vi "cBRS Readout Transfer Function.vi"() -> ()   [LabVIEW 2018]
uses:
  <vilib>/Utility/error.llb/DialogType.ctl
  <vilib>/DAQmx/read.llb/DAQmx Read (Analog 1D Wfm NChan NSamp).vi
  <vilib>/DAQmx/write.llb/DAQmx Write (Analog DBL 1Chan 1Samp).vi
  <vilib>/DAQmx/create/channels.llb/DAQmx Create Channel (AI-Voltage-Basic).vi
  <vilib>/DAQmx/configure/timing.llb/DAQmx Timing (Sample Clock).vi
  <vilib>/DAQmx/create/channels.llb/DAQmx Create Channel (AO-Voltage-Basic).vi
  <vilib>/DAQmx/miscellaneous.llb/DAQmx Fill In Error Info.vi
panel:
  in  "Amplitude":dbl=7.0
  in  "Frequency":dbl
  in  "Capacitor Feedback":bool
  in  "Piezo Feedback":bool
  in  "Gain 1":dbl
  in  "Physical Channel 5":tag="Dev1/ao3" caption="Physical Channel"
  in  "Physical Channel 4":tag="Dev1/ao2" caption="Physical Channel"
  in  "I Reset 2":bool
  in  "I Reset 1":bool
  in  "To Disk Freq":dbl=500.0 caption="dt"
  in  "DC Offset 2":dbl
  in  "I term 2":dbl=5000.0
  in  "Gain 2":dbl=0.005
  in  "Setpoint 2":dbl=5.0
  in  "Physical Channel 3":tag="Dev1/ao1" caption="Physical Channel"
  in  "I term":dbl=5000.0
  in  "Output terminal configuration":i32(ring)=10083 items=["Default"=-1, "RSE"=10083, "Differential"=10106, "Pseudodifferential"=12529]
  in  "DC Offset":dbl
  in  "Gain":dbl=0.005
  in  "Setpoint":dbl=5.0
  in  "Physical Channel 2":tag="Dev1/ao0" caption="Physical Channel"
  in  "Input terminal configuration":i32(ring)=10106 items=["default"=-1, "RSE"=10083, "NRSE"=10078, "Differential"=10106, "Pseudodifferential"=12529]
  in  "Down Sample Freq":dbl=1000.0 caption="dt"
  out "Waveform Chart":dynamicdata(graph)=[{"t0"=timestamp(3662756182.4372287 s since 1904-01-01), "dt"=1.9999999999999998e-05, "Y"=array[500 elements], "attributes"=variant("NI_ChannelName"=variant(string "Dev1/ai0"), "NI_UnitDescription"=variant(string "Volts"))}, {"t0"=timestamp(3662756182.4372387 s since 1904-01-01), "dt"=1.9999999999999998e-05, "Y"=array[500 elements], "attributes"=variant("NI_ChannelName"=variant(string "Dev1/ai2"), "NI_UnitDescription"=variant(string "Volts"))}, {"t0"=timestamp(3662756182.4372287 s since 1904-01-01), "dt"=0.001, "Y"=[0.0, 0.0, 0.0, 0.0, 0.0, 0.0, 0.0, 0.0, 0.0, 0.0], "attributes"=variant("NI_ChannelName"=variant(string "Dev1/ai0 (Filtered)"), "NI_OriginalChannelName"=variant(string "Dev1/ai0"), "NI_UnitDescription"=variant(string "Volts"))}, {"t0"=timestamp(3662756182.4372287 s since 1904-01-01), "dt"=0.001, "Y"=[0.0, 0.0, 0.0, 0.0, 0.0, 0.0, 0.0, 0.0, 0.0, 0.0], "attributes"=variant("NI_ChannelName"=variant(string "Dev1/ai2 (Filtered)"), "NI_OriginalChannelName"=variant(string "Dev1/ai2"), "NI_UnitDescription"=variant(string "Volts"))}, {"t0"=timestamp(3662756182.4372287 s since 1904-01-01), "dt"=0.001, "Y"=[3.746254926547408, 3.7462550457566977, 3.7462551556527615, 3.746255255304277, 3.7462553502991796, 3.746255445294082, 3.7462555365636945, 3.7462556241080165, 3.7462557135149837, 3.7462558085098863], "attributes"=variant("NI_ChannelName"=variant(string "Dev1/ai0 (Filtered)"), "NI_OriginalChannelName"=variant(string "Dev1/ai0"), "NI_UnitDescription"=variant(string "Volts"))}]
  in  "Write":bool caption="Enable"
  in  "stop":bool
  in  "Samples to Read":i32=500
  in  "Sample Rate":dbl=50000.0 caption="Read Rate (Hz)" format="%0.2f"
  in  "Physical Channel":tag="Dev1/ai0, Dev1/ai2" caption="Input Physical Channel"
  # "Piezo Feedback 1"
  # "Piezo Feedback 2"
  # "Capacitor Feedback"
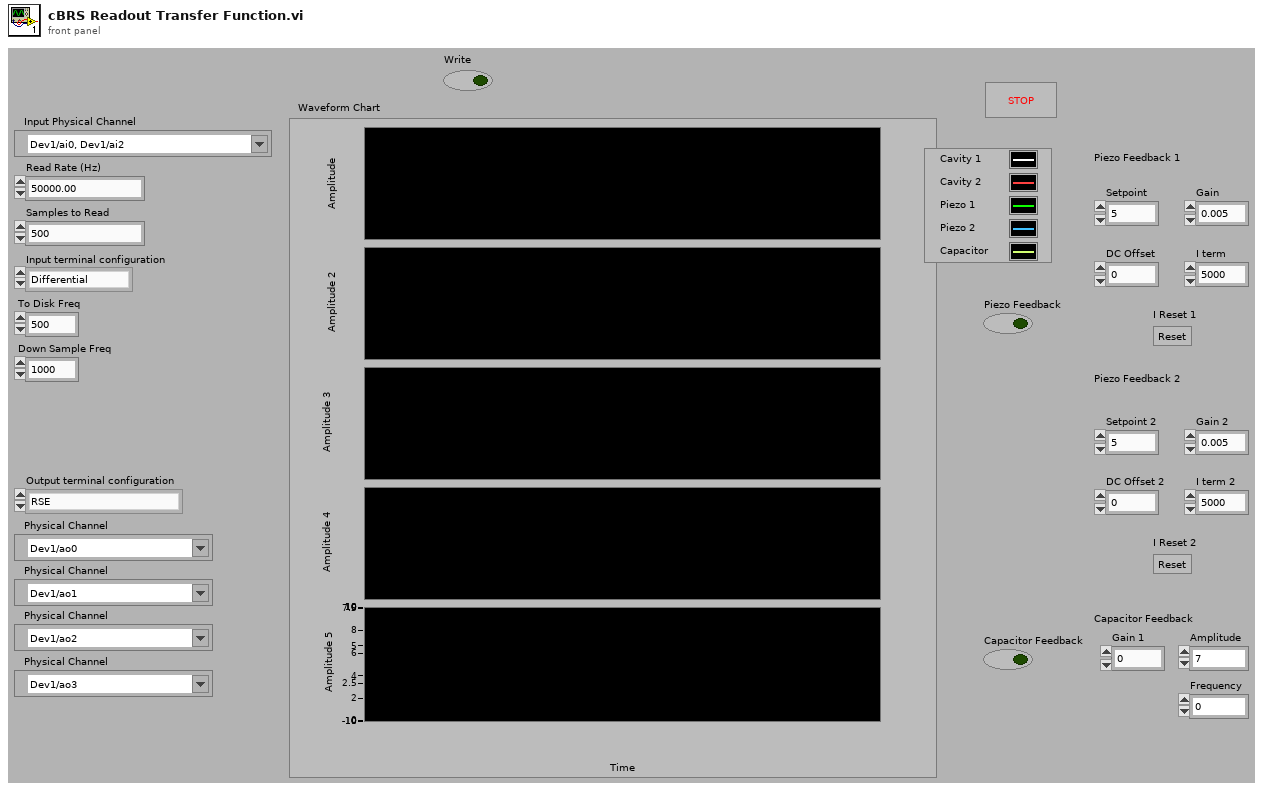
[diagram p1: front panel]
types:
  T1 = typedef "DialogType.ctl" = u16
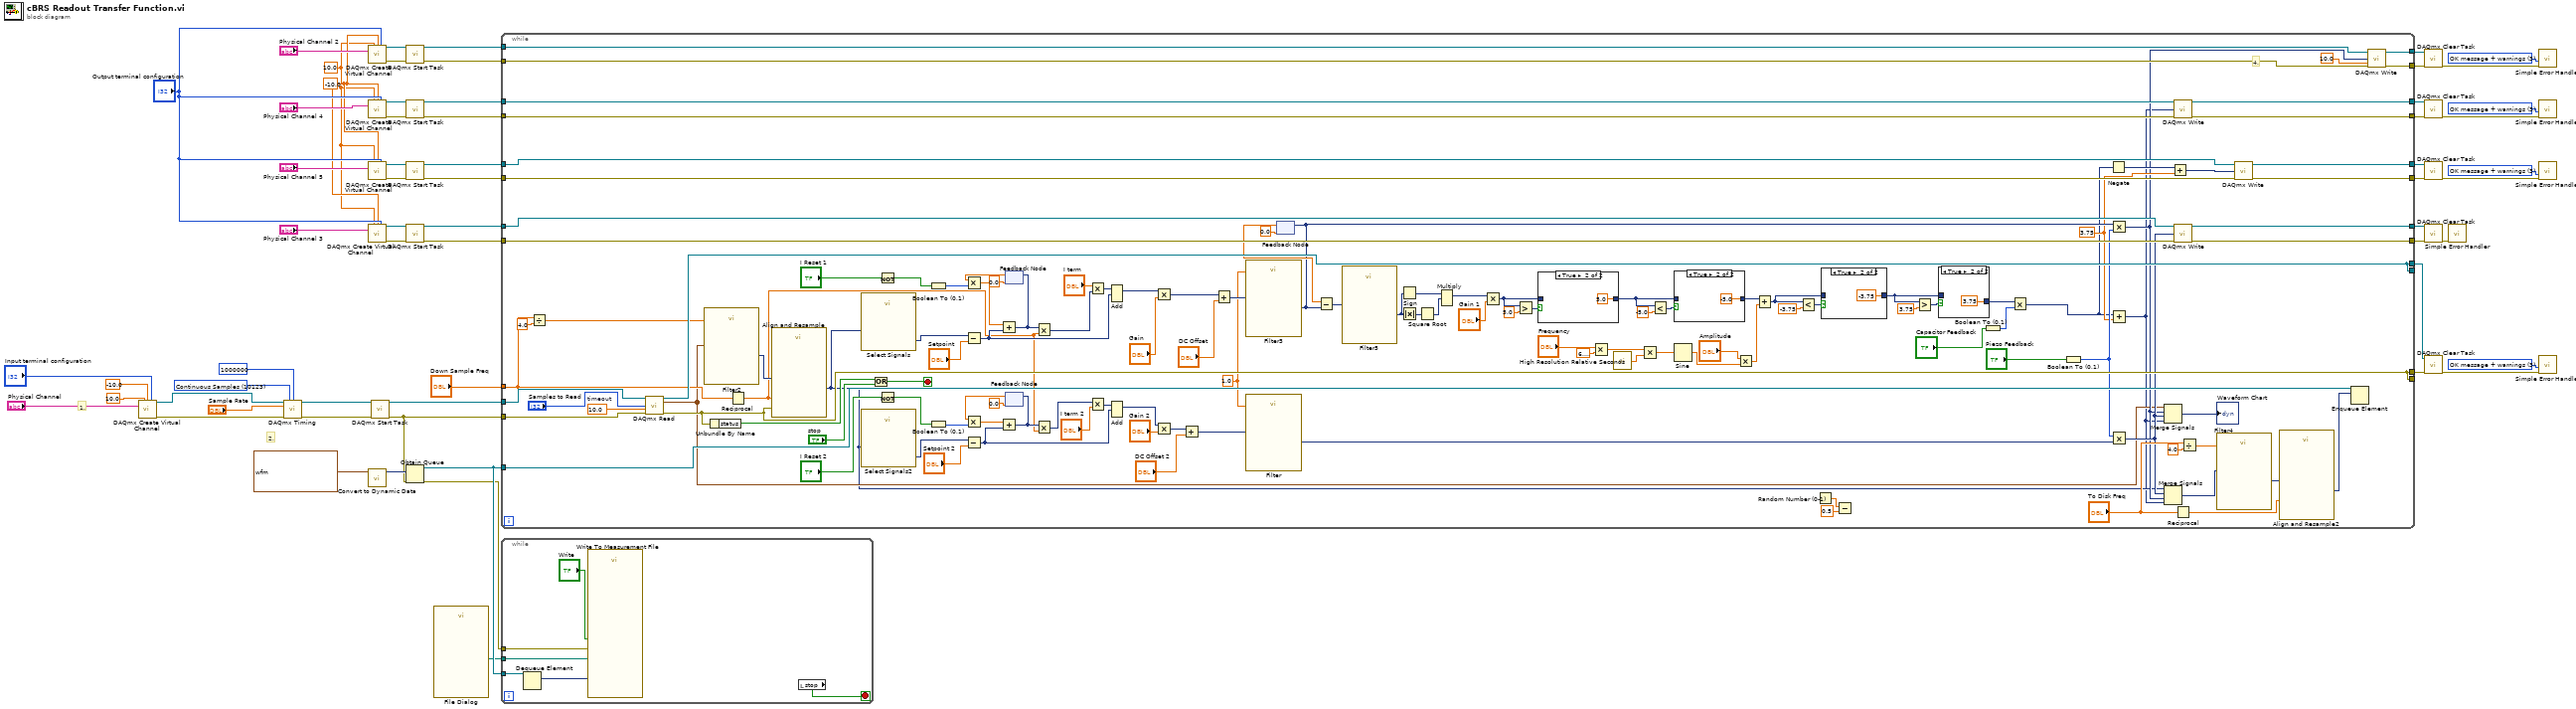
[diagram p0: block diagram]
diagram:
  w2 = 10.0 ("maximum value")
  w3 = -10.0 ("Minimum Value 4")
  w14 = T1 3 items=["no dialog", "OK message", "continue or stop message", "OK message + warnings", "continue/stop + warnings"] ("type of dialog (OK msg:1)")
  w16 = T1 3 items=["no dialog", "OK message", "continue or stop message", "OK message + warnings", "continue/stop + warnings"] ("type of dialog (OK msg:1)")
  w44 = T1 3 items=["no dialog", "OK message", "continue or stop message", "OK message + warnings", "continue/stop + warnings"] ("type of dialog (OK msg:1)")
  w52 = T1 3 items=["no dialog", "OK message", "continue or stop message", "OK message + warnings", "continue/stop + warnings"] ("type of dialog (OK msg:1)")
  w57 = 10123 items=["Finite Samples"=10178, "Continuous Samples"=10123] ("sample mode")
  # "2."
  # "1."
  n1 = call-poly <vilib>:"DAQmx Create Virtual Channel.vi"("maximum value"=10.0, "minimum value"=-10.0 ("Minimum Value"), "input terminal configuration"="Input terminal configuration", "physical channels"="Physical Channel") -> ("task out"=w59:refnum<k21>, "error out"=w61:errorcluster)  [unwired: 10 in]
  n2 = call-poly <vilib>:"DAQmx Timing.vi"("task/channels in"=w59, "sample mode"=w57, "samples per channel"=1000000, "rate"="Sample Rate", "error in"=w61) -> ("task out"=w56:refnum<k21>, "error out"=w55:errorcluster)  [unwired: 9 in]
  n3 = call-poly <vilib>:"DAQmx Create Virtual Channel.vi"("maximum value"=w2, "minimum value"=w3, "output terminal configuration"="Output terminal configuration", "physical channels"="Physical Channel 2") -> ("task out"=w43:refnum<k21>, "error out"=w42:errorcluster)  [unwired: 10 in]
  n4 = call-poly <vilib>:"DAQmx Create Virtual Channel.vi"("maximum value"=w2, "minimum value"=w3, "output terminal configuration"="Output terminal configuration", "physical channels"="Physical Channel 4") -> ("task out"=w23:refnum<k21>, "error out"=w22:errorcluster)  [unwired: 10 in]
  n5 = call-poly <vilib>:"DAQmx Create Virtual Channel.vi"("maximum value"=w2, "minimum value"=w3, "output terminal configuration"="Output terminal configuration", "physical channels"="Physical Channel 5") -> ("task out"=w20:refnum<k21>, "error out"=w19:errorcluster)  [unwired: 10 in]
  n6 = call-poly <vilib>:"DAQmx Create Virtual Channel.vi"("maximum value"=w2, "minimum value"=w3, "output terminal configuration"="Output terminal configuration", "physical channels"="Physical Channel 3") -> ("task out"=w36:refnum<k21>, "error out"=w35:errorcluster)  [unwired: 10 in]
  n7 = call "Convert to Dynamic Data"("Waveform"=waveform(dbl) {"t0"=timestamp(0 s since 1904-01-01), "dt"=1.0, "Y"=[]}) -> ("Dynamic Data Type"=w29:dynamicdata)  [unwired: 3 in]
  n8 = call <vilib>:"DAQmx Start Task.vi"("task/channels in"=w56, "error in"=w55) -> ("task out"=w51:refnum<k21>, "error out"=w27:errorcluster)  [unwired: 12 in]
  n9 = call <vilib>:"DAQmx Start Task.vi"("task/channels in"=w43, "error in"=w42) -> ("task out"=w41:refnum<k21>, "error out"=w40:errorcluster)  [unwired: 12 in]
  n10 = call <vilib>:"DAQmx Start Task.vi"("task/channels in"=w23, "error in"=w22) -> ("task out"=w18:refnum<k21>, "error out"=w9:errorcluster)  [unwired: 12 in]
  n11 = call <vilib>:"DAQmx Start Task.vi"("task/channels in"=w20, "error in"=w19) -> ("task out"=w8:refnum<k21>, "error out"=w7:errorcluster)  [unwired: 12 in]
  n12 = call <vilib>:"DAQmx Start Task.vi"("task/channels in"=w36, "error in"=w35) -> ("task out"=w34:refnum<k21>, "error out"=w33:errorcluster)  [unwired: 12 in]
  n13 = Obtain Queue(element data type=w29, error in (no error)=w27) -> (queue out=w26:refnum<queue>, error out=w25:errorcluster)  [unwired: 3 in, 1 out]
  n14 = call "File Dialog"() -> ("selected path"=w1:path)  [unwired: 12 in, 3 out]
  n15 = while {
    tunnel: w27 -> [w186]
    tunnel: w51 -> [w185]
    tunnel: [w138] -> w50
    tunnel: [w139] -> w54
    tunnel: "Down Sample Freq" -> [w111]
    tunnel: w41 -> [w181]
    tunnel: w40 -> [w180]
    tunnel: [w179] -> w39
    tunnel: [w178] -> w38
    tunnel: w34 -> [w159]
    tunnel: w33 -> [w158]
    tunnel: [w168] -> w32
    tunnel: [w167] -> w30
    tunnel: [w139] -> _
    tunnel: [w138] -> _
    tunnel: w26 -> [w136]
    tunnel: w18 -> [w128]
    tunnel: [w127] -> w13
    tunnel: [w126] -> w12
    tunnel: [w125] -> w11
    tunnel: [w124] -> w10
    tunnel: w9 -> [w123]
    tunnel: w8 -> [w122]
    tunnel: w7 -> [w121]
    stop <- w134 stop-if-true
    w96 = 3.75 ("y")
    w129 = 1.0
    w182 = 10.0  # timeout
    # "4."
    n16 = Divide(x=w111, y=4.0) -> (x/y=w110:dbl)
    n17 = call-poly <vilib>:"DAQmx Read.vi"("task/channels in"=w185, "number of samples per channel"="Samples to Read", "timeout"=w182, "error in"=w186) -> ("task out"=w138:refnum<k21>, "data"=w76:waveform(dbl)[], "error out"=w139:errorcluster)  [unwired: 9 in]
    n18 = call "Filter2"("Lower Cut-Off"=w110, "Signal"=w76) -> ("Filtered Signal"=w174:dynamicdata)  [unwired: 8 in, 1 out]
    n19 = Unbundle By Name(w139) -> ("status"=w184:bool)
    n20 = Reciprocal(x=w111) -> (1/x=w117:dbl)
    n21 = call "Align and Resample"("dt"=w117, "error in (no error)"=w139, "Signals"=w174) -> ("Resampled Signals"=w75:dynamicdata)  [unwired: 6 in, 2 out]
    n22 = call "Select Signals"("Signals"=w75) -> ("Signal Out"=w173:dynamicdata)  [unwired: 9 in, 1 out]
    n23 = call "Select Signals2"("Signals"=w75) -> ("Signal Out"=w137:dynamicdata)  [unwired: 9 in, 1 out]
    n24 = Or(x=w184, y="stop") -> (x .or. y?=w134:bool)
    n25 = Not(x="I Reset 1") -> (.not. x?=w148:bool)
    n26 = Not(x="I Reset 2") -> (.not. x?=w142:bool)
    n27 = Boolean To (0,1)(Boolean=w148) -> (0, 1=w152:i16)
    n28 = Boolean To (0,1)(Boolean=w142) -> (0, 1=w146:i16)
    n29 = Subtract(x=w173, y="Setpoint") -> (x-y=w133:dynamicdata)
    n30 = Subtract(x=w137, y="Setpoint 2") -> (x-y=w132:dynamicdata)
    n31 = feedback #1(0.0) -> (w151:dbl)
    n32 = Multiply(x=w151, y=w152) -> (x*y=w150:dbl)
    n33 = Add(x=w150, y=w133) -> (x+y=w154:dynamicdata)
    n34 = feedback-in #1(w154) -> ()
    n35 = feedback #2(0.0) -> (w145:dbl)
    n36 = Multiply(x=w145, y=w146) -> (x*y=w144:dbl)
    n37 = Add(x=w144, y=w132) -> (x+y=w141:dynamicdata)
    n38 = feedback-in #2(w141) -> ()
    n39 = Multiply(x=w154, y=w117) -> (x*y=w155:dynamicdata)
    n40 = Multiply(x=w141, y=w117) -> (x*y=w140:dynamicdata)
    n41 = Multiply(x="I term", y=w155) -> (x*y=w171:dynamicdata)
    n42 = Multiply(x=w140, y="I term 2") -> (x*y=w164:dynamicdata)
    n43 = Add(1:w133, 2:w171) -> (0:w166:dynamicdata)  [unwired: 1 in, 1 out]
    n44 = Add(1:w132, 2:w164) -> (0:w162:dynamicdata)  [unwired: 1 in, 1 out]
    n45 = Multiply(x=w166, y="Gain") -> (x*y=w157:dynamicdata)
    n46 = Multiply(x=w162, y="Gain 2") -> (x*y=w156:dynamicdata)
    n47 = Add(x=w156, y="DC Offset 2") -> (x+y=w130:dynamicdata)
    n48 = Add(x=w157, y="DC Offset") -> (x+y=w131:dynamicdata)
    n49 = call "Filter3"("Lower Cut-Off"=w129, "Signal"=w131) -> ("Filtered Signal"=w105:dynamicdata)  [unwired: 8 in, 1 out]
    n50 = call "Filter"("Lower Cut-Off"=w129, "Signal"=w130) -> ("Filtered Signal"=w120:dynamicdata)  [unwired: 8 in, 1 out]
    n51 = feedback #3(0.0) -> (w106:dbl)
    n52 = feedback-in #3(w105) -> ()
    n53 = Subtract(x=w106, y=w105) -> (x-y=w104:dynamicdata)
    n54 = call "Filter5"("Signal"=w104) -> ("Filtered Signal"=w100:dynamicdata)  [unwired: 9 in, 1 out]
    n55 = Sign(1:w100) -> (0:w99:dynamicdata)
    n56 = Absolute Value(x=w100) -> (abs(x)=w101:dynamicdata)
    n57 = Square Root(x=w101) -> (sqrt(x)=w98:dynamicdata)
    n58 = Multiply(1:w98, 2:w99) -> (0:w97:dynamicdata)  [unwired: 1 in, 1 out]
    n59 = Multiply(x=w97, y="Gain 1") -> (x*y=w89:dynamicdata)
    n60 = Greater?(x=w89, y=5.0) -> (0:w88:dynamicdata)
    n61 = case shown="True" w88 {
      tunnel: [w193 5.0] -> w86
      tunnel: w89 -> [w193 _]
      frame False {
      }
      frame True {
      }
    }
    n62 = Multiply(x="Frequency", y=6.283185307179586) -> (x*y=w80:dbl)
    n63 = call <vilib>:"High Resolution Relative Seconds.vi"() -> ("relative seconds"=w81:dbl)
    n64 = Multiply(x=w80, y=w81) -> (x*y=w79:dbl)
    n65 = Less?(x=w86, y=-5.0) -> (x < y?=w87:dynamicdata)
    n66 = case shown="True" w87 {
      tunnel: [w191 -5.0] -> w84
      tunnel: w86 -> [w191 _]
      frame False {
      }
      frame True {
      }
    }
    n67 = Sine(x=w79) -> (sin(x)=w63:dbl)
    n68 = Multiply(x="Amplitude", y=w63) -> (x*y=w77:dbl)
    n69 = Add(x=w84, y=w77) -> (x+y=w67:dynamicdata)
    n70 = Less?(x=w67, y=-3.75) -> (x < y?=w74:dynamicdata)
    n71 = Random Number (0-1)() -> (number: 0 to 1=w65:dbl)
    n72 = case shown="True" w74 {
      tunnel: [w189 -3.75] -> w69
      tunnel: w67 -> [w189 _]
      frame False {
      }
      frame True {
      }
    }
    n73 = Subtract(x=w65, y=0.5) -> ()  [unwired: 1 out]
    n74 = Greater?(x=w69, y=3.75) -> (0:w71:dynamicdata)
    n75 = case shown="True" w71 {
      tunnel: [w187 3.75] -> w70
      tunnel: w69 -> [w187 _]
      frame False {
      }
      frame True {
      }
    }
    n76 = Boolean To (0,1)(Boolean="Capacitor Feedback") -> (0, 1=w94:i16)
    n77 = Multiply(x=w70, y=w94) -> (x*y=w62:dynamicdata)
    n78 = Boolean To (0,1)(Boolean="Piezo Feedback") -> (0, 1=w109:i16)
    n79 = Negate(x=w62) -> (-x=w95:dynamicdata)
    n80 = Multiply(x=w105, y=w109) -> (x*y=w92:dynamicdata)
    n81 = Add(x=w62, y=w96) -> (x+y=w64:dynamicdata)
    n82 = Multiply(x=w109, y=w120) -> (x*y=w93:dynamicdata)
    n83 = Merge Signals(w76, w92, w93, w64) -> (→"Waveform Chart":dynamicdata)
    n84 = Merge Signals(w75, w93, w92, w64) -> (w91:dynamicdata)
    n85 = Add(x=w95, y=w96) -> (x+y=w68:dynamicdata)
    n86 = call-poly <vilib>:"DAQmx Write.vi"("task/channels in"=w128, "data"=w64, "error in"=w123) -> ("task out"=w124:refnum<k21>, "error out"=w125:errorcluster)  [unwired: 10 in, 1 out]
    n87 = call-poly <vilib>:"DAQmx Write.vi"("task/channels in"=w159, "data"=w93, "error in"=w158) -> ("task out"=w167:refnum<k21>, "error out"=w168:errorcluster)  [unwired: 10 in, 1 out]
    n88 = Reciprocal(x="To Disk Freq") -> (1/x=w118:dbl)
    n89 = Divide(x="To Disk Freq", y=4.0) -> (x/y=w113:dbl)
    n90 = call "Filter4"("Lower Cut-Off"=w113, "Signal"=w91) -> ("Filtered Signal"=w116:dynamicdata)  [unwired: 8 in, 1 out]
    n91 = call-poly <vilib>:"DAQmx Write.vi"("task/channels in"=w122, "data"=w68, "error in"=w121) -> ("task out"=w127:refnum<k21>, "error out"=w126:errorcluster)  [unwired: 10 in, 1 out]
    n92 = call "Align and Resample2"("dt"=w118, "Signals"=w116) -> ("Resampled Signals"=w135:dynamicdata)  [unwired: 7 in, 2 out]
    n93 = Enqueue Element(queue=w136, element=w135) -> ()  [unwired: 2 in, 3 out]
    n94 = call-poly <vilib>:"DAQmx Write.vi"("task/channels in"=w181, "data"=w92, "timeout"=10.0, "error in"=w180) -> ("task out"=w178:refnum<k21>, "error out"=w179:errorcluster)  [unwired: 9 in, 1 out]
  }
  n95 = while {
    tunnel: w26 -> [w200]
    tunnel: w25 -> [w197]
    tunnel: w1 -> [w195]
    stop <- w198 stop-if-true
    n96 = Dequeue Element(queue=w200) -> (element=w199:dynamicdata)  [unwired: 2 in, 3 out]
    n97 = call "Write To Measurement File"("Signals"=w199, "Enable"="Write", "error in (no error)"=w197, "Filename"=w195) -> ()  [unwired: 13 in, 3 out]
    n98 = local read "stop"() -> (w198:bool)
  }
  n99 = call <vilib>:"DAQmx Clear Task.vi"("task in"=w38, "error in"=w39) -> ("error out"=w46:errorcluster)  [unwired: 13 in]
  n100 = call <vilib>:"DAQmx Clear Task.vi"("task in"=w10, "error in"=w11) -> ("error out"=w17:errorcluster)  [unwired: 13 in]
  n101 = call <vilib>:"DAQmx Clear Task.vi"("task in"=w13, "error in"=w12) -> ("error out"=w15:errorcluster)  [unwired: 13 in]
  n102 = call <vilib>:"DAQmx Clear Task.vi"("task in"=w30, "error in"=w32) -> ("error out"=w31:errorcluster)  [unwired: 13 in]
  n103 = call <vilib>:"DAQmx Clear Task.vi"("task in"=w50, "error in"=w54) -> ("error out"=w60:errorcluster)  [unwired: 13 in]
  n104 = call <vilib>:"Simple Error Handler.vi"("error in (no error)"=w31) -> ()  [unwired: 4 in, 5 out]
  n105 = call <vilib>:"Simple Error Handler.vi"("type of dialog (OK msg:1)"=w44, "error in (no error)"=w46) -> ()  [unwired: 3 in, 5 out]
  n106 = call <vilib>:"Simple Error Handler.vi"("type of dialog (OK msg:1)"=w16, "error in (no error)"=w17) -> ()  [unwired: 3 in, 5 out]
  n107 = call <vilib>:"Simple Error Handler.vi"("type of dialog (OK msg:1)"=w14, "error in (no error)"=w15) -> ()  [unwired: 3 in, 5 out]
  n108 = call <vilib>:"Simple Error Handler.vi"("type of dialog (OK msg:1)"=w52, "error in (no error)"=w60) -> ()  [unwired: 3 in, 5 out]
